vi "Keithley 2002 2-W Res Config.vi"(0 "GPIB address":string="16", 1 "range value (ohms)":dbl=1000000000.0 min=20.0 max=1000000000.0 format="%^.2e", 2 "range (auto:0)":u16(ring) items=["autorange", "autorange once", "set min range", "set max range", "set range value"], 3 "dig. filter count":dbl=10.0 min=1.0 max=100.0 step=1.0 format="%^.2e", 4 "digital filter (off:0)":u16(ring) items=["off", "auto filter", "auto filter once", "moving filter", "repeating filter"], 5 "integration time (0:auto)":u16(ring) items=["automatic", "automatic once", "set to minimum", "set to maximum", "set aperature value", "set NPLC value"], 7 "integ. value":dbl=0.01667 format="%^.2e", 8 "advanced filter (off:0)":u16(ring) items=["off", "enabled"], 9 "resolution (4.5 digits:3)":u16(ring)=3 items=["auto resolution", "auto resolution once", "3.5 digits", "4.5 digits", "5.5 digits", "6.5 digits", "7.5 digits", "8.5 digits", "8.5 digits", "8.5 digits"], 10 "noise tolerance (%)":dbl=1.0 min=0.0 max=100.0 step=1.0 format="%^.2e", 11 "error in":T1, 12 "reference (off:0)":u16(ring) items=["off", "set reference value"], 13 "reference value (ohms)":dbl min=-1000000000.0 max=1000000000.0 format="%^.2e", 14 "offset compensation":bool) -> (15 "error out":T1)   [LabVIEW 2020]
doc: "This VI is used to configure the settings for the 2-wire resistance measurements. The instrument can be any mode when this VI is run. The settings will go into effect and the instrument will enter the 2-wire resistance mode."
panel:
  # "on\noff"
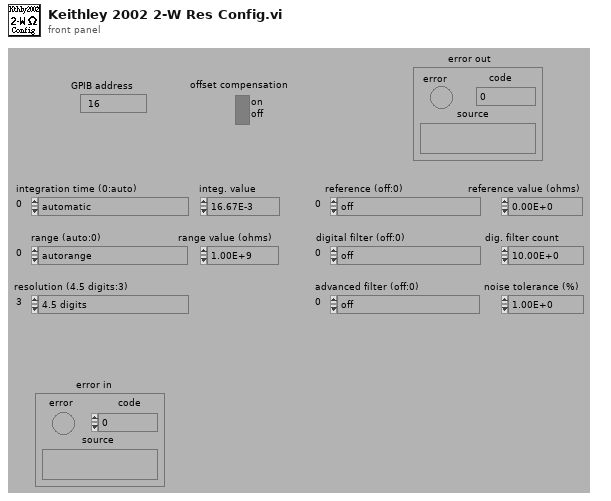
[diagram p1: front panel]
types:
  T1 = cluster{"error":bool, "code":i32, "source":string}
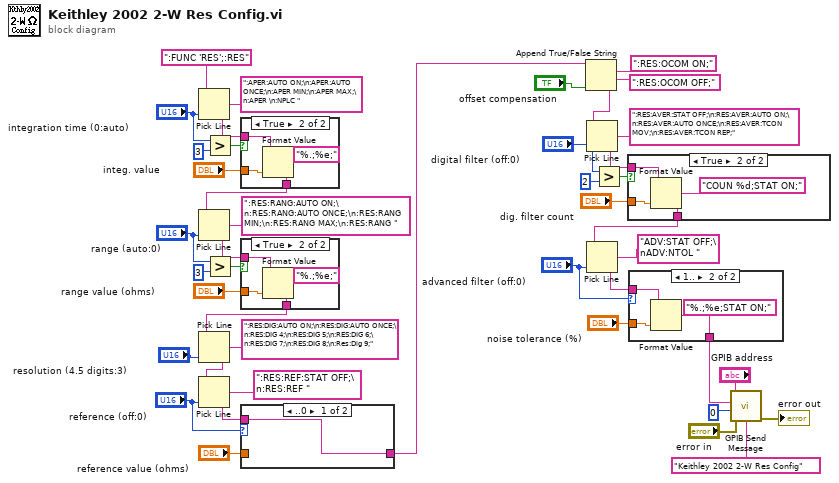
[diagram p0: block diagram]
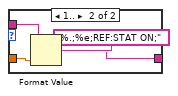
[diagram p4: hidden frame]
diagram:
  n1 = Pick Line(string ("")=":FUNC 'RES';:RES", multi-line string=":APER:AUTO ON;\n:APER:AUTO ONCE;\n:APER MIN;\n:APER MAX;\n:APER \n:NPLC ", line index="integration time (0:auto)") -> (output string=w38:string)
  n2 = Greater?(x="integration time (0:auto)", y=3) -> (0:w39:bool)
  n3 = Greater?(x="range (auto:0)", y=3) -> (0:w36:bool)
  n4 = case shown="True" w39 {
    tunnel: "integ. value" -> [_ w48]
    tunnel: w38 -> [w45 w47]
    tunnel: [w45 w46] -> w31
    frame False {
    }
    frame True {
      n5 = Format Value(string ("")=w47, format string="%.;%e;", value (0)=w48) -> (output string=w46:string)
    }
  }
  n6 = Pick Line(string ("")=w31, multi-line string=":RES:RANG:AUTO ON;\n:RES:RANG:AUTO ONCE;\n:RES:RANG MIN;\n:RES:RANG MAX;\n:RES:RANG ", line index="range (auto:0)") -> (output string=w37:string)
  n7 = case shown="True" w36 {
    tunnel: "range value (ohms)" -> [_ w53]
    tunnel: w37 -> [w50 w52]
    tunnel: [w50 w51] -> w28
    frame False {
    }
    frame True {
      n8 = Format Value(string ("")=w52, format string="%.;%e;", value (0)=w53) -> (output string=w51:string)
    }
  }
  n9 = Pick Line(string ("")=w28, multi-line string=":RES:DIG:AUTO ON;\n:RES:DIG:AUTO ONCE;\n:RES:DIG 4;\n:RES:DIG 5;\n:RES:DIG 6;\n:RES:DIG 7;\n:RES:DIG 8;\n:Res:Dig 9;", line index="resolution (4.5 digits:3)") -> (output string=w24:string)
  n10 = Pick Line(string ("")=w24, multi-line string=":RES:REF:STAT OFF;\n:RES:REF ", line index="reference (off:0)") -> (output string=w27:string)
  n11 = case shown="..0" "reference (off:0)" {
    tunnel: "reference value (ohms)" -> [_ w59]
    tunnel: w27 -> [w55 w58]
    tunnel: [w55 w56] -> w1
    frame ..0 {
    }
    frame 1.. {
      n12 = Format Value(string ("")=w58, format string="%.;%e;REF:STAT ON;", value (0)=w59) -> (output string=w56:string)
    }
  }
  n13 = Append True/False String(1:"offset compensation", 2:":RES:OCOM OFF;", 3:":RES:OCOM ON;", 4:w1) -> (0:w5:string)
  n14 = Pick Line(string ("")=w5, multi-line string=":RES:AVER:STAT OFF;\n:RES:AVER:AUTO ON;\n:RES:AVER:AUTO ONCE;\n:RES:AVER:TCON MOV;\n:RES:AVER:TCON REP;", line index="digital filter (off:0)") -> (output string=w21:string)
  n15 = Greater?(x="digital filter (off:0)", y=2) -> (0:w18:bool)
  n16 = case shown="True" w18 {
    tunnel: "dig. filter count" -> [_ w64]
    tunnel: w21 -> [w60 w63]
    tunnel: [w60 w62] -> w10
    frame False {
    }
    frame True {
      n17 = Format Value(string ("")=w63, format string="COUN %d;STAT ON;", value (0)=w64) -> (output string=w62:string)
    }
  }
  n18 = Pick Line(string ("")=w10, multi-line string="ADV:STAT OFF;\nADV:NTOL ", line index="advanced filter (off:0)") -> (output string=w14:string)
  n19 = case shown="1.." "advanced filter (off:0)" {
    tunnel: "noise tolerance (%)" -> [_ w69]
    tunnel: w14 -> [w65 w68]
    tunnel: [w65 w67] -> w11
    frame ..0 {
    }
    frame 1.. {
      n20 = Format Value(string ("")=w68, format string="%.;%e;STAT ON;", value (0)=w69) -> (output string=w67:string)
    }
  }
  n21 = call "GPIB Send Message.vi"("address string"="GPIB address", "write buffer"=w11, "source"="Keithley 2002 2-W Res Config", "write mode (set END:0)"=0, "error in"="error in") -> ("error out"=→"error out":T1)  [unwired: 2 in, 2 out]
